vi "Decode Signal Patterns.vi"(11 "Signal Pattern":string[](array[string])) -> (3 "Segment Pattern":string[](array[string]))   [LabVIEW 2021]
panel:
  out "Seg4":string
  out "Seg6":string
  out "Seg5":string
  out "Seg7":string
  out "Seg3":string
  out "Seg2":string
  out "Seg1":string
  out "Signal Length":i32[](array[numeric])
  out "Character Count":cluster{string, i32}[](array[cluster])
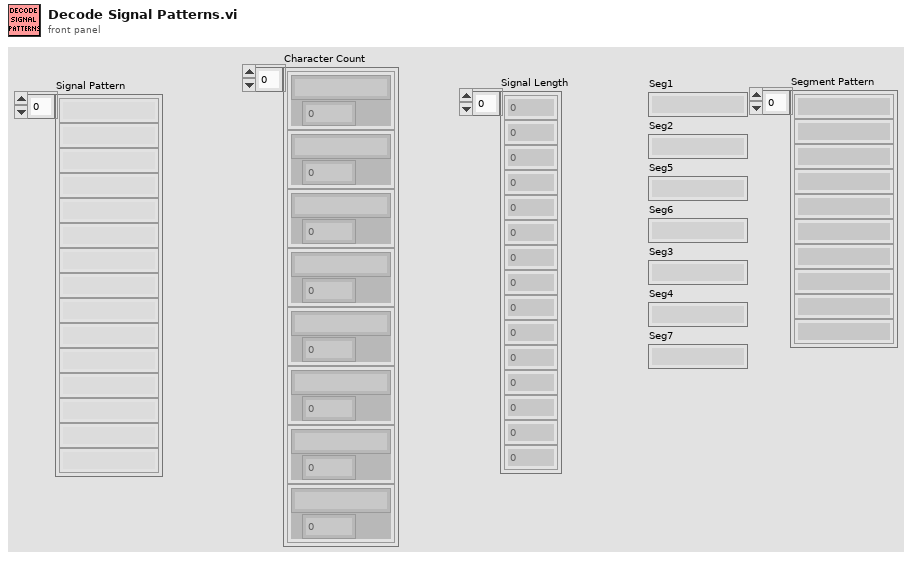
[diagram p1: front panel]
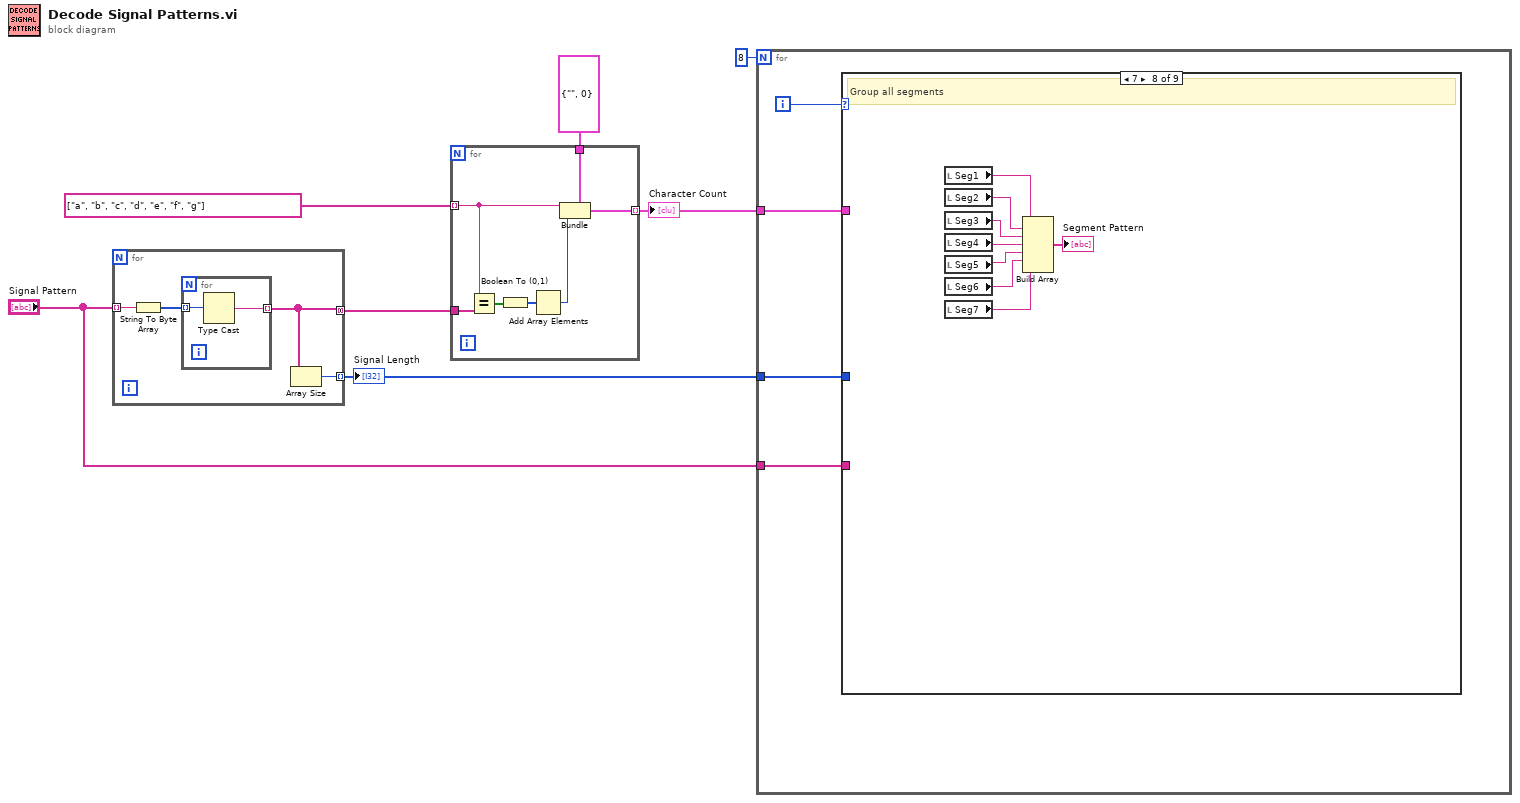
[diagram p0: block diagram]
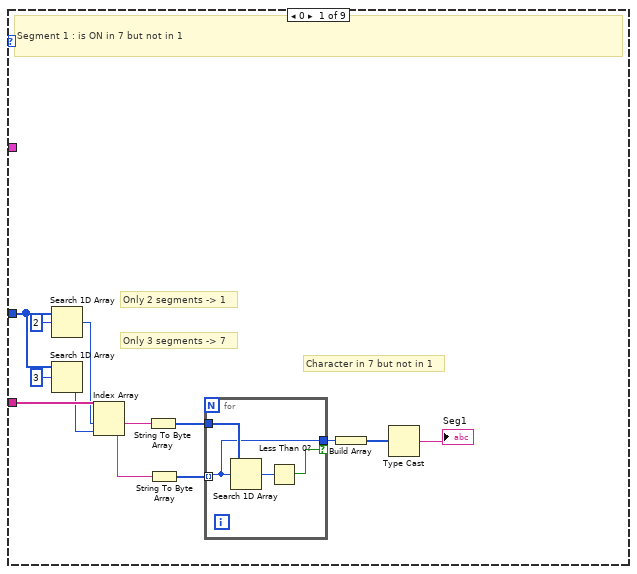
[diagram p2: hidden frame]
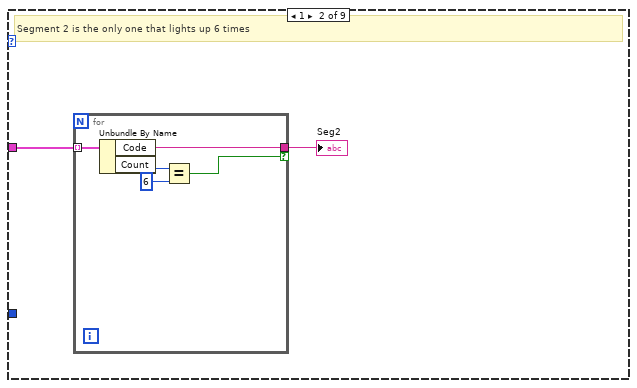
[diagram p3: hidden frame]
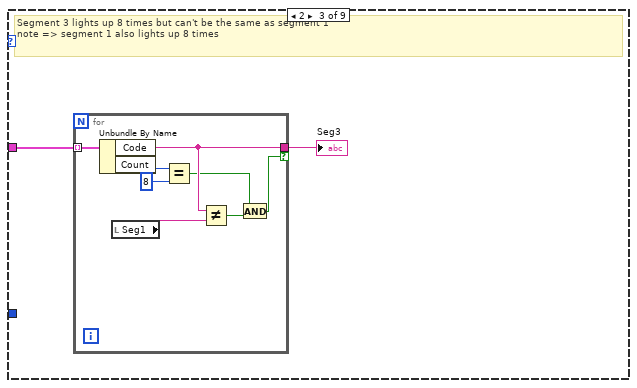
[diagram p4: hidden frame]
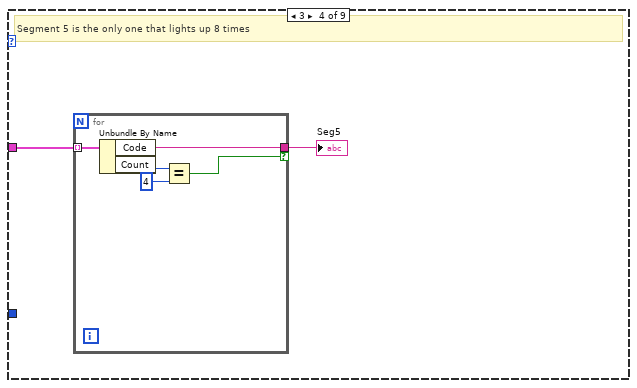
[diagram p5: hidden frame]
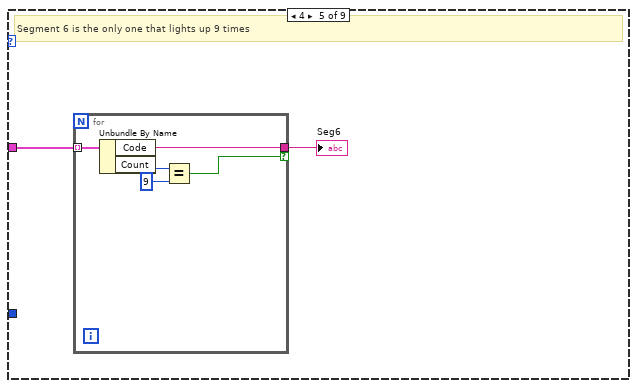
[diagram p6: hidden frame]
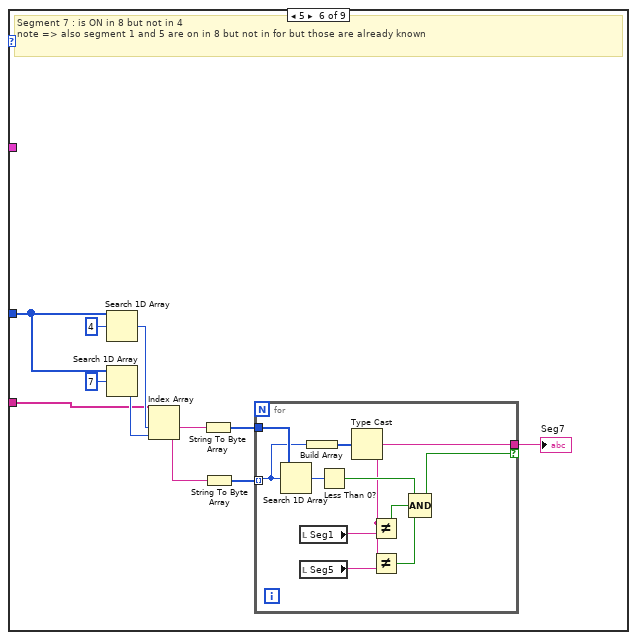
[diagram p7: hidden frame]
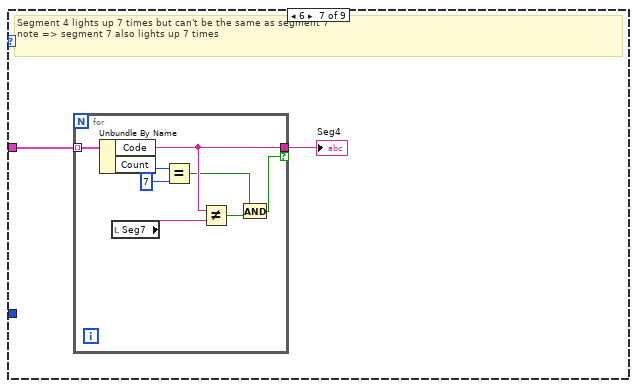
[diagram p8: hidden frame]
diagram:
  n1 = for {
    tunnel: "Signal Pattern" -> [w11] mode=indexing
    tunnel: [w9] -> w7 mode=concatenating
    tunnel: [w8] -> w4 mode=indexing
    n2 = String To Byte Array(string=w11) -> (unsigned byte array=w10:u8[])
    n3 = for {
      tunnel: w10 -> [w13] mode=indexing
      tunnel: [w12] -> w9 mode=indexing
      n4 = Type Cast(x=w13) -> (*(type *) &x=w12:string)  [unwired: 1 in]
    }
    n5 = Array Size(array=w9) -> (size(s)=w8:i32)
  }
  "Signal Length" <- w4
  n6 = for {
    tunnel: w7 -> [w18]
    tunnel: string[] ["a", "b", "c", "d", "e", "f", "g"] -> [w17] mode=indexing
    tunnel: [w20] -> w2 mode=indexing
    tunnel: cluster{"Code":string, "Count":i32} {"Code"="", "Count"=0} -> [w19]
    n7 = Equal?(x=w17, y=w18) -> (x = y?=w16:bool[])
    n8 = Boolean To (0,1)(Boolean=w16) -> (0, 1=w15:i16[])
    n9 = Add Array Elements(numeric array=w15) -> (sum=w14:i16)
    n10 = Bundle(cluster=w19, "Code"=w17, "Count"=w14) -> (w20:cluster{"Code":string, "Count":i32})
  }
  "Character Count" <- w2
  n11 = for {
    N: 8 -> [_]
    tunnel: w4 -> [w23]
    tunnel: "Signal Pattern" -> [w22]
    tunnel: w2 -> [w21]
    i -> [w24]
    n12 = case shown="7" w24 {
      tunnel: w23 -> [w35 _ _ _ _ w77 _ _ _]
      tunnel: w22 -> [w34 _ _ _ _ w76 _ _ _]
      tunnel: w21 -> [_ w43 w50 w60 w67 _ w96 _ _]
      frame 0 {
        # "Character in 7 but not in 1"
        # "Only 3 segments -> 7"
        # "Only 2 segments -> 1"
        # "Segment 1 : is ON in 7 but not in 1"
        n13 = Search 1D Array(1D array=w35, element=2) -> (index of element=w32:i32)  [unwired: 1 in]
        n14 = Search 1D Array(1D array=w35, element=3) -> (index of element=w33:i32)  [unwired: 1 in]
        n15 = Index Array(array=w34, index #1=w32, index #2=w33) -> (element #1=w31:string, element #2=w30:string)
        n16 = String To Byte Array(string=w31) -> (unsigned byte array=w29:u8[])
        n17 = String To Byte Array(string=w30) -> (unsigned byte array=w28:u8[])
        n18 = for {
          tunnel: w29 -> [w40]
          tunnel: w28 -> [w39] mode=indexing
          tunnel: [w39] -> w27 if=w38
          n19 = Search 1D Array(1D array=w40, element=w39) -> (index of element=w41:i32)  [unwired: 1 in]
          n20 = Less Than 0?(x=w41) -> (x < 0?=w38:bool)
        }
        n21 = Build Array(w27) -> (w26:u8[])
        n22 = Type Cast(x=w26) -> (*(type *) &x=→"Seg1":string)  [unwired: 1 in]
      }
      frame 1 {
        # "Segment 2 is the only one that lights up 6 times"
        n23 = for {
          tunnel: w43 -> [w48] mode=indexing
          tunnel: [w45] -> w42 if=w44
          n24 = Unbundle By Name(w48) -> ("Code"=w45:string, "Count"=w47:i32)
          n25 = Equal?(x=w47, y=6) -> (x = y?=w44:bool)
        }
        "Seg2" <- w42
      }
      frame 2 {
        # "Segment 3 lights up 8 times but can't be the same as segment 1\nnote => segment 1 also lights up 8 times"
        n26 = for {
          tunnel: w50 -> [w58] mode=indexing
          tunnel: [w55] -> w49 if=w52
          n27 = Unbundle By Name(w58) -> ("Code"=w55:string, "Count"=w57:i32)
          n28 = local read "Seg1"() -> (w51:string)
          n29 = Equal?(x=w57, y=8) -> (x = y?=w53:bool)
          n30 = Not Equal?(x=w55, y=w51) -> (x != y?=w54:bool)
          n31 = And(x=w53, y=w54) -> (x .and. y?=w52:bool)
        }
        "Seg3" <- w49
      }
      frame 3 {
        # "Segment 5 is the only one that lights up 8 times"
        n32 = for {
          tunnel: w60 -> [w65] mode=indexing
          tunnel: [w62] -> w59 if=w61
          n33 = Unbundle By Name(w65) -> ("Code"=w62:string, "Count"=w64:i32)
          n34 = Equal?(x=w64, y=4) -> (x = y?=w61:bool)
        }
        "Seg5" <- w59
      }
      frame 4 {
        # "Segment 6 is the only one that lights up 9 times"
        n35 = for {
          tunnel: w67 -> [w72] mode=indexing
          tunnel: [w69] -> w66 if=w68
          n36 = Unbundle By Name(w72) -> ("Code"=w69:string, "Count"=w71:i32)
          n37 = Equal?(x=w71, y=9) -> (x = y?=w68:bool)
        }
        "Seg6" <- w66
      }
      frame 5 {
        # "Segment 7 : is ON in 8 but not in 4\nnote => also segment 1 and 5 are on in 8 but not in for but those are already known"
        n38 = Search 1D Array(1D array=w77, element=4) -> (index of element=w80:i32)  [unwired: 1 in]
        n39 = Search 1D Array(1D array=w77, element=7) -> (index of element=w81:i32)  [unwired: 1 in]
        n40 = Index Array(array=w76, index #1=w80, index #2=w81) -> (element #1=w79:string, element #2=w78:string)
        n41 = String To Byte Array(string=w79) -> (unsigned byte array=w75:u8[])
        n42 = String To Byte Array(string=w78) -> (unsigned byte array=w74:u8[])
        n43 = for {
          tunnel: w75 -> [w93]
          tunnel: w74 -> [w92] mode=indexing
          tunnel: [w84] -> w73 if=w87
          n44 = Search 1D Array(1D array=w93, element=w92) -> (index of element=w94:i32)  [unwired: 1 in]
          n45 = local read "Seg1"() -> (w89:string)
          n46 = local read "Seg5"() -> (w86:string)
          n47 = Build Array(w92) -> (w91:u8[])
          n48 = Less Than 0?(x=w94) -> (x < 0?=w90:bool)
          n49 = Type Cast(x=w91) -> (*(type *) &x=w84:string)  [unwired: 1 in]
          n50 = Not Equal?(x=w84, y=w89) -> (x != y?=w88:bool)
          n51 = Not Equal?(x=w84, y=w86) -> (x != y?=w85:bool)
          n52 = Compound Arithmetic op=AND(w90, w88, w85) -> (w87:bool)
        }
        "Seg7" <- w73
      }
      frame 6 {
        # "Segment 4 lights up 7 times but can't be the same as segment 7\nnote => segment 7 also lights up 7 times"
        n53 = for {
          tunnel: w96 -> [w104] mode=indexing
          tunnel: [w101] -> w95 if=w98
          n54 = Unbundle By Name(w104) -> ("Code"=w101:string, "Count"=w103:i32)
          n55 = local read "Seg7"() -> (w97:string)
          n56 = Equal?(x=w103, y=7) -> (x = y?=w99:bool)
          n57 = Not Equal?(x=w101, y=w97) -> (x != y?=w100:bool)
          n58 = And(x=w99, y=w100) -> (x .and. y?=w98:bool)
        }
        "Seg4" <- w95
      }
      frame 7 {
        # "Group all segments"
        n59 = local read "Seg1"() -> (w111:string)
        n60 = local read "Seg2"() -> (w110:string)
        n61 = local read "Seg3"() -> (w109:string)
        n62 = local read "Seg4"() -> (w112:string)
        n63 = local read "Seg5"() -> (w108:string)
        n64 = local read "Seg6"() -> (w107:string)
        n65 = local read "Seg7"() -> (w106:string)
        n66 = Build Array(w111, w110, w109, w112, w108, w107, w106) -> (→"Segment Pattern":string[])
      }
      frame Default {
      }
    }
  }
